vi "Get EL-RIO-CM PIDs.vi"() -> (3 "EL-RIO-CM PIDs":u32[](array[numeric]) format="%.0x")   [LabVIEW 2021]
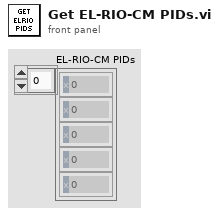
[diagram p1: front panel]
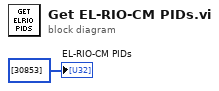
[diagram p0: block diagram]
diagram:
  "EL-RIO-CM PIDs" <- u32[] [30853]
